vi "My_Dual Channel PID.vi"() -> ()   [LabVIEW 2018]
doc: "This example demonstrates how to create a dual PID controller."
uses:
  <vilib>/addons/control/pid/pid.llb/PID (DBL).vi
  <vilib>/addons/control/pid/NI_PID_pid.lvlib
panel:
  in  "Load (%) 2":dbl(slide)=88.0 scale=0.0..100.0
  in  "Load (%)":dbl(slide)=58.0 scale=0.0..100.0
  in  "derivative time (Td, min) 2":dbl format="%.3f"
  in  "integral time (Ti, min) 2":dbl=0.056 format="%.3f"
  in  "proportional gain (Kc) 2":dbl=50.0 format="%.3f"
  in  "derivative time (Td, min)":dbl=0.001 format="%.3f"
  in  "integral time (Ti, min)":dbl=0.1 format="%.3f"
  in  "proportional gain (Kc)":dbl=50.0 format="%.3f"
  in  "Gain 1":dbl(slide)=3.2203389830508473 scale=0.0..5.0
  in  "Gain 2":dbl(slide)=2.642857142857143 scale=0.0..5.0
  in  "SP2:":dbl(slide)=35.294117647058826 min=0.0 max=0.0 scale=0.0..100.0
  out "MV2:":dbl(slide)=100.0 scale=-100.0..100.0
  out "PV2:":dbl(slide)=19.422100390987225 scale=0.0..100.0
  in  "SP1:":dbl(slide)=60.7843137254902 min=0.0 max=0.0 scale=0.0..100.0
  out "MV1:":dbl(slide)=100.0 scale=-100.0..100.0
  out "PV1:":dbl(slide)=29.253567073551352 scale=0.0..100.0
  in  "Sampling Time dt (s)":dbl=0.05 min=0.001 step=0.01 format="%#.3p"
  in  "Stop":bool
  out "Process Variable and Setpoint":T1(graph)={"initial PV"=29.253567073551352, "SP1:"=60.7843137254902, "initial PV"=19.422100390987225, "SP2:"=35.294117647058826}
  # "Overview: This example demonstrates how to create a dual PID controller.\nInstructions:\n1. Run the VI and observe the Process Variable (PV) following the Setpoint (SP) for both Controllers.\n2. Change the setpoint of one controller and verify that it does not affect the second controller.\n3. Click Stop to stop the VI."
  # "PID Parameters"
  # "Plants Parameters"
  # "Controller 1"
  # "Controller 2"
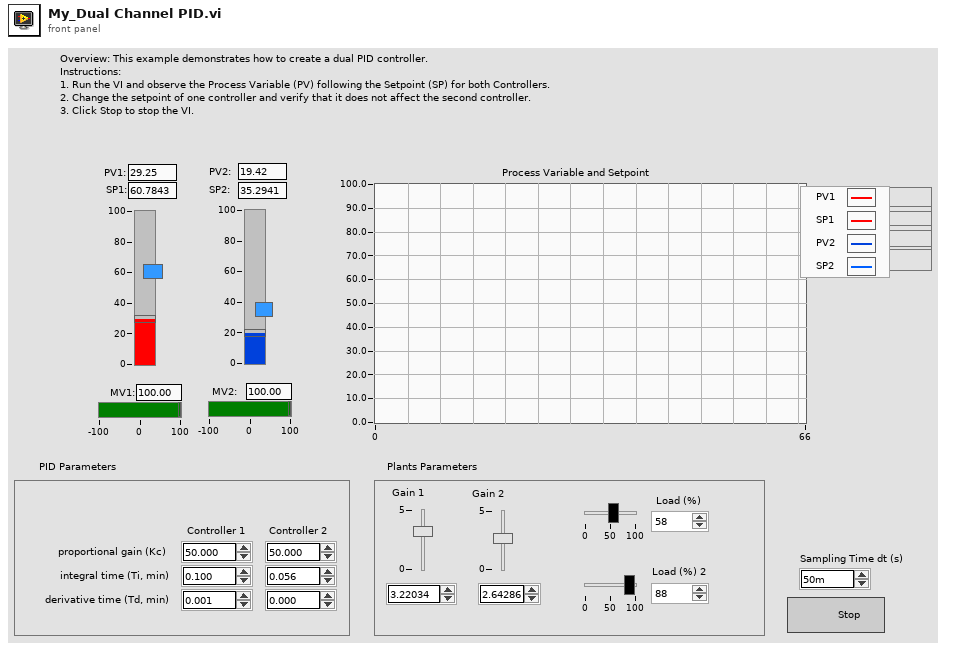
[diagram p1: front panel]
types:
  T1 = cluster{"initial PV":dbl, "SP1:":dbl, "initial PV":dbl, "SP2:":dbl}
  T2 = cluster{"static gain":dbl, "lag (min)":dbl, "dead cycles":dbl, "load %":dbl, "deadband":dbl, "noise level %":dbl, "initial PV":dbl, "initial PV 2":dbl}
  T3 = cluster{"proportional gain (Kc)":dbl, "integral time (Ti, min)":dbl, "derivative time (Td, min)":dbl}
  T4 = cluster{"proportional gain (Kc) 2":dbl, "integral time (Ti, min) 2":dbl, "derivative time (Td, min) 2":dbl}
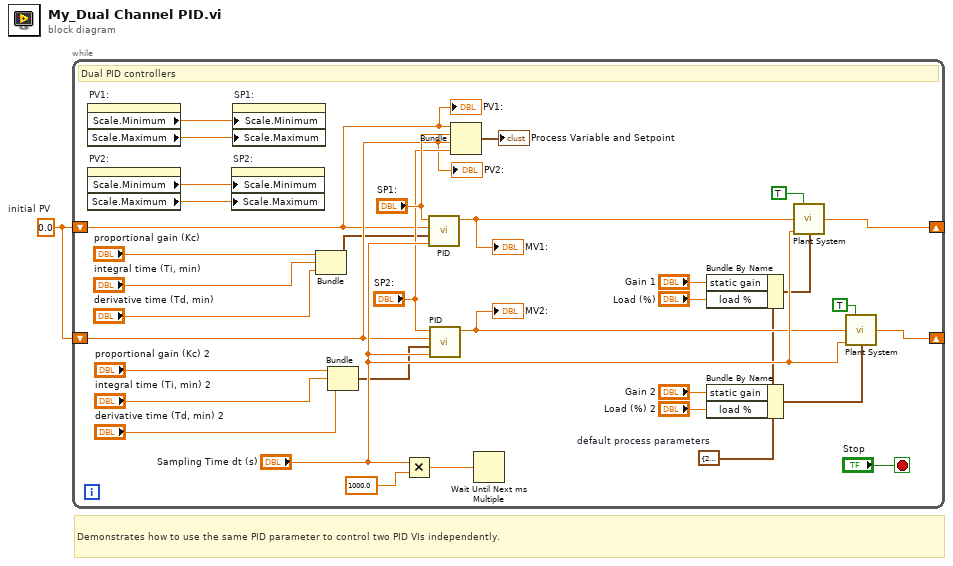
[diagram p0: block diagram]
diagram:
  w1 = 0.0  # initial PV
  # "Demonstrates how to use the same PID parameter to control two PID VIs independently."
  n1 = while {
    shift-left: w1 -> [w21]
    shift-right: [w31] -> _
    shift-right: [w27] -> _
    shift-left: w1 -> [w22]
    stop <- "Stop" stop-if-true
    w7 = T2 {"static gain"=2.5, "lag (min)"=18.0, "dead cycles"=0.0, "load %"=40.0, "deadband"=2.0, "noise level %"=0.25, "initial PV"=0.0, "initial PV 2"=0.0}  # default process parameters
    # "Dual PID controllers"
    n2 = property on="PV1:" class="Slide (strict)"() -> ("Scale.Minimum"=w30:dbl, "Scale.Maximum"=w29:dbl)  [unwired: 2 in, 2 out]
    n3 = property on="PV2:" class="Slide (strict)"() -> ("Scale.Minimum"=w25:dbl, "Scale.Maximum"=w24:dbl)  [unwired: 2 in, 2 out]
    n4 = property on="SP2:" class="Slide (strict)"("Scale.Minimum"=w25, "Scale.Maximum"=w24) -> ()  [unwired: 2 in, 2 out]
    n5 = property on="SP1:" class="Slide (strict)"("Scale.Minimum"=w30, "Scale.Maximum"=w29) -> ()  [unwired: 2 in, 2 out]
    n6 = Bundle("proportional gain (Kc)"="proportional gain (Kc)", "integral time (Ti, min)"="integral time (Ti, min)", "derivative time (Td, min)"="derivative time (Td, min)") -> (w17:T3)  [unwired: 1 in]
    n7 = Bundle("proportional gain (Kc) 2"="proportional gain (Kc) 2", "integral time (Ti, min) 2"="integral time (Ti, min) 2", "derivative time (Td, min) 2"="derivative time (Td, min) 2") -> (w13:T4)  [unwired: 1 in]
    n8 = Multiply(x="Sampling Time dt (s)", y=1000.0) -> (x*y=w3:dbl)
    n9 = call-poly <vilib>:"PID.vi"("dt (s)"="Sampling Time dt (s)", "PID gains"=w17, "process variable"=w21, "setpoint"="SP1:") -> ("output"=w33:dbl)  [unwired: 6 in, 1 out]
    "MV1:" <- w33
    n10 = call-poly <vilib>:"PID.vi"("dt (s)"="Sampling Time dt (s)", "PID gains"=w13, "process variable"=w22, "setpoint"="SP2:") -> ("output"=w26:dbl)  [unwired: 6 in, 1 out]
    "MV2:" <- w26
    n11 = Bundle("initial PV"=w21, "SP1:"="SP1:", "initial PV"=w22, "SP2:"="SP2:") -> (→"Process Variable and Setpoint":T1)  [unwired: 1 in]
    n12 = Wait Until Next ms Multiple(millisecond multiple=w3) -> ()  [unwired: 1 out]
    n13 = Bundle By Name(cluster=w7, "static gain"="Gain 1", "load %"="Load (%)") -> (w10:T2)
    n14 = Bundle By Name(cluster=w7, "static gain"="Gain 2", "load %"="Load (%) 2") -> (w6:T2)
    n15 = call "Plant System.vi"("Integrator ?"=TRUE, "Plant Input"=w33, "dt (s)"="Sampling Time dt (s)", "process parameters"=w10) -> ("Plant Output"=w31:dbl)  [unwired: 11 in]
    n16 = call "Plant System.vi"("Integrator ?"=TRUE, "Plant Input"=w26, "dt (s)"="Sampling Time dt (s)", "process parameters"=w6) -> ("Plant Output"=w27:dbl)  [unwired: 11 in]
    "PV1:" <- w21
    "PV2:" <- w22
  }
